vi "Convert RPM to CTRE Encoder Velocity.vi"(10 "Units/ Rev":dbl, 11 "RPM":dbl) -> (3 "CTRE Vel (units/.1S) Out":dbl)   [LabVIEW 2020, in "Shooter_ACT.lvlib"]
uses:
  Shooter_ACT.lvlib
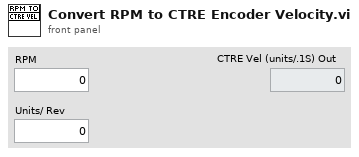
[diagram p1: front panel]
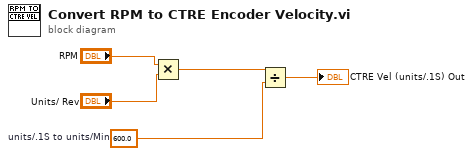
[diagram p0: block diagram]
diagram:
  w2 = 600.0  # units/.1S to units/Min
  n1 = Multiply(x="RPM", y="Units/ Rev") -> (x*y=w1:dbl)
  n2 = Divide(x=w1, y=w2) -> (x/y=→"CTRE Vel (units/.1S) Out":dbl)
